vi "AppendString.vi"(0 ".NET Refnum":refnum<k24>, 1 "String To Append":string) -> (2 ".NET Refnum Out":refnum<k24>, 3 "String Out":string, 4 "error out":errorcluster)   [LabVIEW 2013]
uses:
  C:/perforce/TestStand/Tests/LVBuildValidation/13.0/Automated/FlexLVAdapter30/Refnums/DotNetRefnum/LabviewDNTest.dll
  LabviewDNTest.dll
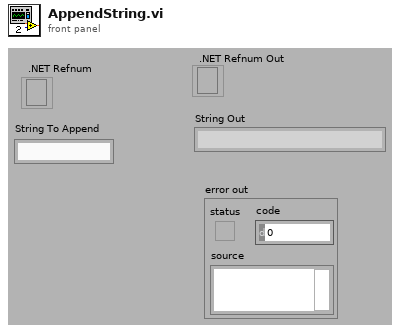
[diagram p1: front panel]
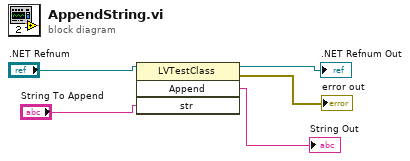
[diagram p0: block diagram]
diagram:
  n1 = invoke class="LVTestClass" method="Append"(reference=".NET Refnum", "str"="String To Append") -> (reference out=→".NET Refnum Out":refnum<k24>, error out=→"error out":errorcluster, "Append"=→"String Out":string)  [unwired: 2 in, 1 out]
